vi "Set Timeout.vi"(8 "error in (no error)":errorcluster caption="entrée d'erreur (pas d'erreur)", 10 "Timeout":u32, 11 "Class Balance (Default) en entrée":refnum<class "Class Balance (Default).lvclass">) -> (0 "error out":errorcluster caption="sortie d'erreur", 3 "Class Balance (Default) en sortie":refnum<class "Class Balance (Default).lvclass">)   [LabVIEW 2020, in "Library Instrument & Equipement.lvlib" / "Library Balance.lvlib" / "Class Balance (Default).lvclass"]
uses:
  Class Balance (Default).lvclass
  Class Balance (Default).lvclass/Class Balance (Default).ctl
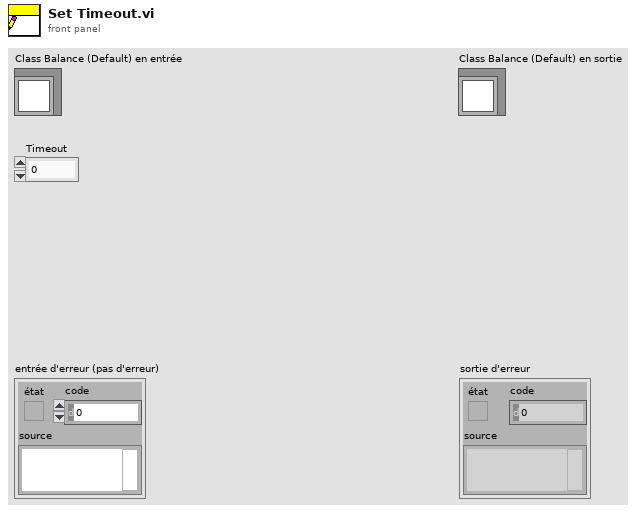
[diagram p1: front panel]
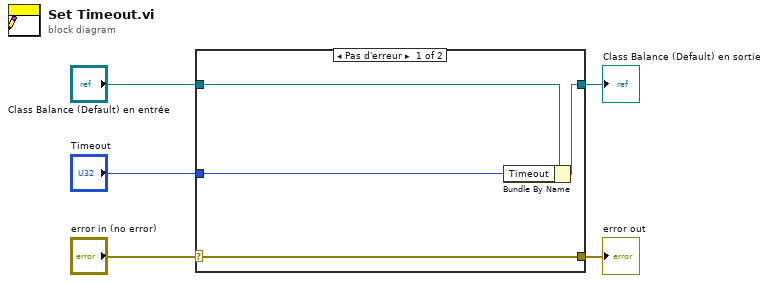
[diagram p0: block diagram]
diagram:
  n1 = case shown="Pas d'erreur" "error in (no error)" {
    selector: "error in (no error)" -> [w9 w10]
    tunnel: [w9 w10] -> w4
    tunnel: [w7 w11] -> w2
    tunnel: "Class Balance (Default) en entrée" -> [w8 w11]
    tunnel: "Timeout" -> [w6 _]
    frame No Error {
      n2 = Bundle By Name(cluster=w8, "Timeout"=w6) -> (w7:refnum<class "Class Balance (Default).lvclass">)
    }
    frame Error {
    }
  }
  "error out" <- w4
  "Class Balance (Default) en sortie" <- w2
